vi "changeErrorCode.vi"(8 "error in (no error)":errorcluster, 10 "?":i32, 11 "Model in":refnum<class "Model.lvclass">) -> (0 "error out":errorcluster, 3 "Model out":refnum<class "Model.lvclass">)   [LabVIEW 2016, in "Model.lvclass"]
doc: "Updates the values of the error code and publishes the new value."
uses:
  Model.lvclass
  Typedefs/PubDataSignals.ctl
  Typedefs/SEDSpectrometerTypedefs.lvlib
  ts_sallv_FiberSpectrograph/DataTypes/logevent_errorCode.ctl
  ts_sallv_FiberSpectrograph/SALLV_FiberSpectrograph.lvlib
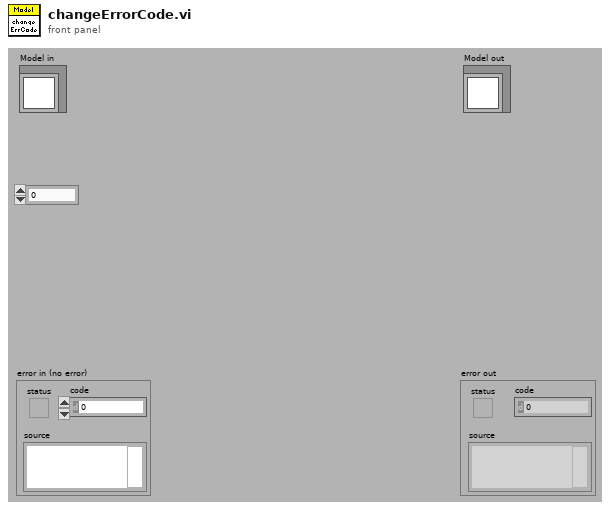
[diagram p1: front panel]
types:
  T1 = typedef "SALLV_FiberSpectrograph.lvlib/logevent_errorCode.ctl" = cluster{"errorCode":i32, "priority":i32}
  T2 = typedef "SEDSpectrometerTypedefs.lvlib/PubDataSignals.ctl" = enum16{"DetailedState", "ErrorCode", "Heartbeat", "LoopTime_ms", "LoopTimeOutOfRange", "RejectedCommand", "SummaryState", "Timestamp", "SettingVersions", "AppliedSettingsMatchStart", "TimeOut", "MeasuredSpectrum", "LargeFileObjectAvailable"}
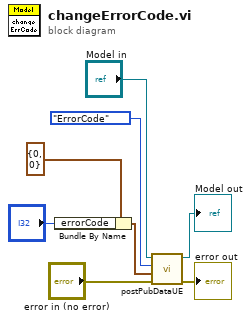
[diagram p0: block diagram]
diagram:
  n1 = Bundle By Name(cluster=T1 {"errorCode"=0, "priority"=0} ("event data"), "errorCode"="?") -> (w1:T1)
  n2 = call "postPubDataUE.vi"("error in (no error)"="error in (no error)", "value"=w1, "pubDataSV"=PubDataSignals."ErrorCode", "Model in"="Model in") -> ("error out"=→"error out":errorcluster, "Model out"=→"Model out":refnum<class "Model.lvclass">)  [unwired: 6 in]
